vi "1.vi"() -> ()   [LabVIEW 2019]
uses:
  <vilib>/Utility/file.llb/Read Delimited Spreadsheet (DBL).vi
panel:
  in  "Path":path
  out "Waveform Chart":dbl(graph)
  out "a+b":dbl
  in  "b":dbl
  in  "a":dbl
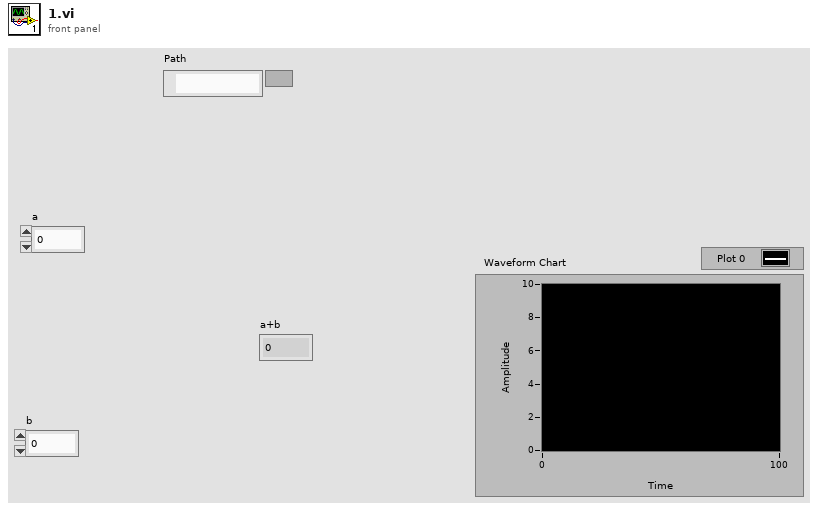
[diagram p1: front panel]
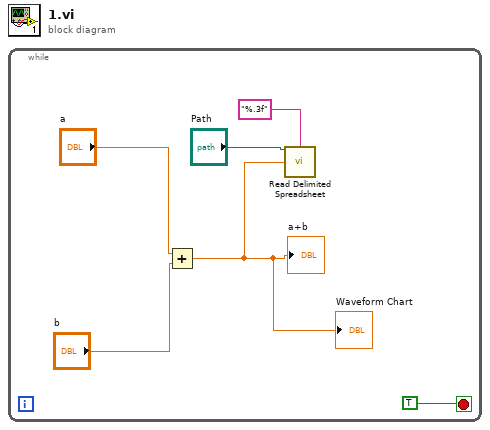
[diagram p0: block diagram]
diagram:
  n1 = while {
    stop <- TRUE stop-if-true
    n2 = Add(x="a", y="b") -> (x+y=w2:dbl)
    "a+b" <- w2
    "Waveform Chart" <- w2
    n3 = call-poly <vilib>:"Read Delimited Spreadsheet.vi"("file path (dialog if empty)"="Path", "format (%.3f)"="%.3f", "start of read offset (chars.:0)"=w2) -> ()  [unwired: 7 in, 6 out]
  }
